vi "setSheetNameByIndex.vi"(8 "error in (no error)":errorcluster, 9 "Sheet Name":string, 10 "Sheet Index":i32, 11 "MS-Excel in":refnum<class "MS-Excel.lvclass">) -> (0 "error out":errorcluster, 3 "MS-Excel out":refnum<class "MS-Excel.lvclass">)   [LabVIEW 2017, in "LabVIEW NPOI.lvlib" / "MS-Excel.lvclass"]
uses:
  MS-Excel.lvclass
  MS-Excel.lvclass/MS-Excel.ctl
  C:/Users/Neo/Desktop/Dev_Tools_BR/LabVIEW_NPOI/lib/NPOI 2.1.1/NPOI.dll
  lib/NPOI 2.1.1/NPOI.dll
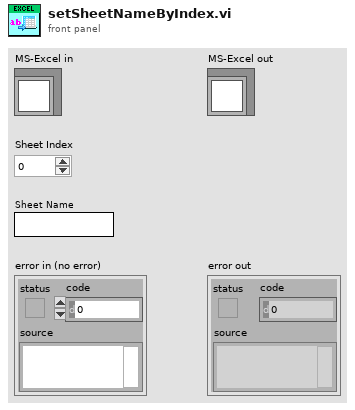
[diagram p1: front panel]
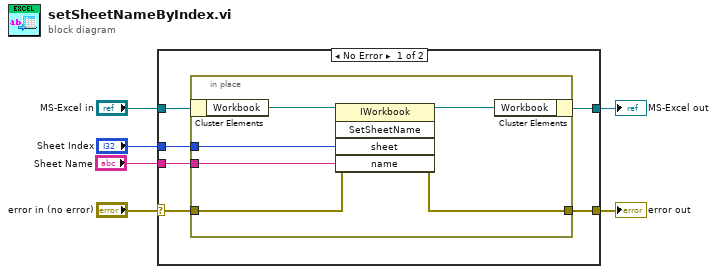
[diagram p0: block diagram]
diagram:
  n1 = case shown="No Error" "error in (no error)" {
    selector: "error in (no error)" -> [w9 w19]
    tunnel: [w8 w19] -> w6
    tunnel: [w12 w20] -> w4
    tunnel: "MS-Excel in" -> [w11 w20]
    tunnel: "Sheet Index" -> [w10 _]
    tunnel: "Sheet Name" -> [w7 _]
    frame No Error {
      n2 = in-place {
        in-place-border: w10 -> [w16]
        in-place-border: w9 -> [w15]
        in-place-border: [w14] -> w8
        in-place-border: w7 -> [w13]
        n3 = in-place-cluster #1(w11) -> ("Workbook"=w18:refnum<k24>)
        n4 = invoke class="IWorkbook" method="SetSheetName"(reference=w18, error in=w15, "sheet"=w16, "name"=w13) -> (reference out=w17:refnum<k24>, error out=w14:errorcluster)  [unwired: 1 in, 3 out]
        n5 = in-place-cluster #1("Workbook"=w17) -> (w12:refnum<class "MS-Excel.lvclass">)
      }
    }
    frame Error {
    }
  }
  "error out" <- w6
  "MS-Excel out" <- w4
